vi "TryUpdateDigitalOutputSample.vi"   [LabVIEW 2018]
uses:
  <vilib>/Platform/TimedLoop/XDataNode/timing_clust.ctl
  <vilib>/Platform/TimedLoop/XDataNode/nitl_modes.ctl
  <vilib>/Platform/TimedLoop/XDataNode/wakeup.ctl
  Telemetry/TelemetryDataTypes.ctl
  Telemetry/TelemetryUpdateModes.ctl
  Telemetry/TelemetryFields.ctl
  <vilib>/rvi/Emulation/niFpgaEmulationIsFPGAContextNoSignature.vi
  <vilib>/rvi/Emulation/niFpgaSctlEmulationGetInTimedLoop.vi
  <vilib>/rvi/errors/niFpgaSetErrorForExecOnDevCompSimple.vi
  <vilib>/rvi/eio/common/nirviEmuReportErrorAndStop.vi
  <vilib>/rvi/DataTransferAndStorage/Container/Common/niFpgaContainerGetUniqueNameForEmu.vi
  <vilib>/rvi/FIFO/Fifo_Resource/nirvififoEmulationSetSize.vi
  <vilib>/rvi/FIFO/Fifo_Resource/nirviFifoEmulationQueueMgr.vi
  <instcachedir>/0/nirviFifoEmulationQueueMgr_E5CAEC123FF24DC58D834DCA3CDAA9B5.lvgen/nirviFifoEmulationQueueMgr_E5CAEC123FF24DC58D834DCA3CDAA9B5_013.vi
  <vilib>/Utility/error.llb/Clear Errors.vi
  <vilib>/rvi/FIFO/Fifo_Resource/nirvififoEmulationCreateLock.vi
  <vilib>/rvi/Emulation/niFpgaProcessEmulError.vi
  <vilib>/rvi/FIFO/Fifo_Resource/nirvififoEmulationObtainLock.vi
  <vilib>/rvi/FIFO/Fifo_Resource/nirvififoEmulationReleaseLock.vi
  <vilib>/rvi/occurrence/nirviWaitOnOccurrenceBase.vi
  <vilib>/rvi/errors/nirviReportUnexpectedCaseInternalError.vi
  <vilib>/rvi/errors/nirviReportUnexpectedCaseInternalError (U32).vi
  <vilib>/rvi/Emulation/niFpgaEmulationReportErrorSimple.vi
  <vilib>/rvi/Emulation/niFpgaGetClockAttributes.vi
  <vilib>/rvi/Emulation/niFpgaCriticalErrorInLSC.vi
  <instcachedir>/0/nirviFifoEmulationQueueMgr_E5CAEC123FF24DC58D834DCA3CDAA9B5.lvgen/nirviFifoEmulationQueueMgr_E5CAEC123FF24DC58D834DCA3CDAA9B5_007.vi
  <vilib>/rvi/FIFO/Fifo_Resource/nirvififoEmulationDetermineInputValidOut.vi
  <vilib>/rvi/Memory/Memory_Emulation/niFpgaMemoryEmulationCacheClearOnFirstRun.vi
  <vilib>/rvi/Memory/Memory_Emulation/nirvimemoryEmulationManagerCache_MakeExclusive.vi
  <vilib>/rvi/Memory/Memory_Emulation/niFpgaMemoryEmulationValidateCache.vi
  <vilib>/rvi/Memory/Memory_Emulation/nirvimemoryEmulationManagerCache_InsertValue.vi
  <vilib>/rvi/Memory/Memory_Emulation/nirvimemoryEmulationManagerCache_ReleaseExclusive.vi
  <vilib>/rvi/Memory/Memory_Emulation/nirvimemoryEmulationManagerCache_GetValue.vi
  <vilib>/rvi/Memory/Memory_Emulation/nirvimemoryEmulationManagerCache_SetValue.vi
  <instcachedir>/0/nirviFifoEmulationQueueMgr_E5CAEC123FF24DC58D834DCA3CDAA9B5.lvgen/nirviFifoEmulationQueueMgr_E5CAEC123FF24DC58D834DCA3CDAA9B5_002.vi
  <vilib>/rvi/DataTransferAndStorage/Container/XNode/niFpgaContainer.xnode
  <vilib>/rvi/FIFO/Fifo_Resource/nirvififoEmulationRead.vi
  <vilib>/Platform/TimedLoop/XDataNode/XDataNode.xnode
  <vilib>/rvi/FIFO/Fifo_Resource/nirvififoEmulationWrite.vi
  <vilib>/rvi/DataTransferAndStorage/Register/Emulation/niFpgaRegisterEmulation.vi
  <vilib>/Platform/TimedLoop/XDataNode/XDNodeRunTimeDep.lvlib
types:
  T1 = cluster{"Sample":u64, "Timestamp":u64, "Value":u16}
  T2 = typedef "TelemetryFields.ctl" = enum16{"None", "InclinometerTxBytes", "InclinometerRxBytes", "InclinometerTxFrames", "InclinometerRxFrames", "InclinometerErrorTimestamp", "InclinometerErrorCode", "InclinometerSampleTimestamp", "InclinometerAngleRaw", "DisplacementTxBytes", "DisplacementRxBytes", "DisplacementTxFrames", "DisplacementRxFrames", "DisplacementErrorTimestamp", "DisplacementErrorCode", "DisplacementSampleTimestamp", "DisplacementRaw1", "DisplacementRaw2", "DisplacementRaw3", "DisplacementRaw4", "DisplacementRaw5", "DisplacementRaw6", "DisplacementRaw7", "DisplacementRaw8", "AccelerometerSampleCount", "AccelerometerSampleTimestamp", "AccelerometerRaw1", "AccelerometerRaw2", "AccelerometerRaw3", "AccelerometerRaw4", "AccelerometerRaw5", "AccelerometerRaw6", "AccelerometerRaw7", "AccelerometerRaw8", "GyroTxBytes", "GyroRxBytes", "GyroTxFrames", "GyroRxFrames", "GyroErrorTimestamp", "GyroErrorCode", "GyroSampleTimestamp", "GyroRawX", "GyroRawY", "GyroRawZ", "GyroStatus", "GyroSequenceNumber", "GyroTemperature", "GyroBITTimestamp", "GyroBIT0", "GyroBIT1", "GyroBIT2", "GyroBIT3", "GyroBIT4", "GyroBIT5", "GyroBIT6", "GyroBIT7", "DigitalInputSampleCount", "DigitalInputTimestamp", "DigitalInputStates", "DigitalOutputSampleCount", "DigitalOutputTimestamp", "DigitalOutputStates", "PowerSupplySampleCount", "PowerSupplyTimestamp", "PowerSupplyStates", "Modbus1ErrorFlags", "Modbus1TxByteCount", "Modbus1TxFrameCount", "Modbus1RxByteCount", "Modbus1RxFrameCount", "Modbus2ErrorFlags", "Modbus2TxByteCount", "Modbus2TxFrameCount", "Modbus2RxByteCount", "Modbus2RxFrameCount", "Modbus3ErrorFlags", "Modbus3TxByteCount", "Modbus3TxFrameCount", "Modbus3RxByteCount", "Modbus3RxFrameCount", "Modbus4ErrorFlags", "Modbus4TxByteCount", "Modbus4TxFrameCount", "Modbus4RxByteCount", "Modbus4RxFrameCount"}
  T3 = typedef "TelemetryUpdateModes.ctl" = enum8{"=", "+", "-", "|"}
  T4 = typedef "TelemetryDataTypes.ctl" = enum8{"U8", "U16", "U32", "U64", "I8", "I16", "I32", "I64", "SGL"}
  T5 = typedef "XDNodeRunTimeDep.lvlib/timing_clust.ctl" = cluster{"Expected End [f-1]":u64, "Actual End [f-1]":u64, "Finished Late? [f-1]":bool, "Expected End [i-1]":u64, "Actual End [i-1]":u64, "Finished Late? [i-1]":bool, "Expected Start [i]":u64, "Actual Start [i]":u64, "Expected Start [f]":u64, "Actual Start [f]":u64, "Source Name":string, "Structure Name":string, "Period":i64, "Deadline":i64, "Offset":i64, "Start":i64, "Priority":i32, "Timeout":i32, "Mode":T6, "Wakeup Reason":T7, "Error":errorcluster, "Source Type":string, "Secondary Source Type":string, "Global End Time":u64, "Global Start Time":u64, "Frame Duration":u64, "Iteration Duration":u64, "Assigned CPU":i32, "I/O Scan Engine Mode":u32}
  T6 = typedef "XDNodeRunTimeDep.lvlib/nitl_modes.ctl" = enum32{"No Change", "Process missed periods, maintain original phase", "Discard missed periods, maintain original phase", "Process missed periods, ignore original phase", "Discard missed periods, ignore original phase"}
  T7 = typedef "XDNodeRunTimeDep.lvlib/wakeup.ctl" = enum32{"Normal", "Aborted", "Asynchronous wakeup", "Timing source error", "Timed loop error", "Timeout"}
  T8 = typedef "TelemetryUpdateData.ctl" = cluster{"DataType":T4, "Mode":T3, "Field":T2, "Data":u64}
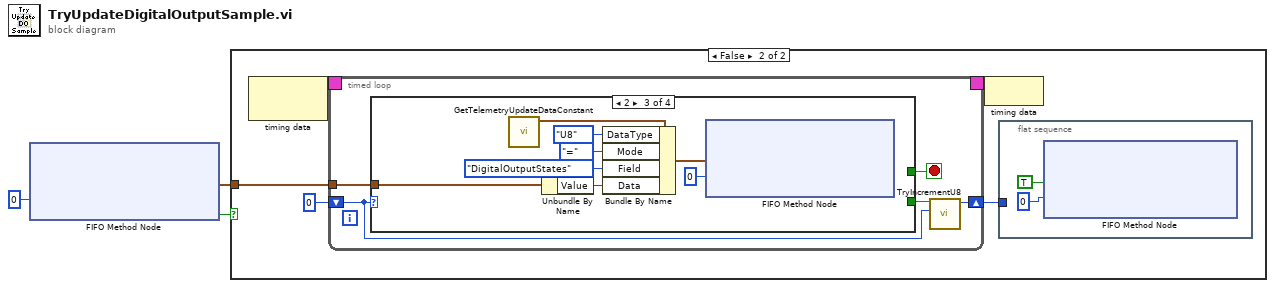
[diagram p0: block diagram]
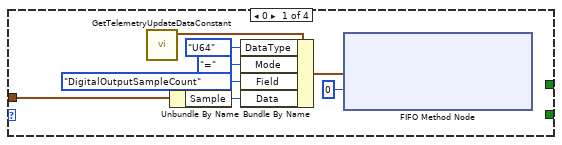
[diagram p3: hidden frame]
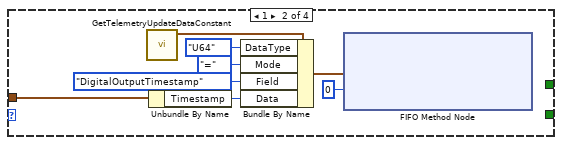
[diagram p4: hidden frame]
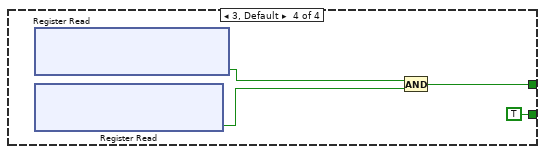
[diagram p5: hidden frame]
diagram:
  n1 = xnode ("FIFO Method Node")("Timeout"=0) -> ("Element"=w2:T1, "Timed Out?"=w3:bool)  [unwired: 1 in, 1 out]
  n2 = case shown="False" w3 {
    tunnel: w2 -> [_ w8]
    frame True {
    }
    frame False {
      n3 = node-c288() -> (w7:T5)  [unwired: 1 in]
      n4 = timed-loop {
        tunnel: w8 -> [w13]
        timing: w7 -> [_]
        timing-out: [_] -> w6
        shift-right: [w11] -> w4
        shift-left: u8 0 -> [w10]
        stop <- w12 stop-if-true
        # "Move Data to Memory"
        n5 = case shown="2" w10 {
          tunnel: w13 -> [w15 w23 w31 _]
          tunnel: [_ _ _ w41] -> w12
          tunnel: [_ _ _ TRUE] -> w9
          frame 0 {
            n6 = call "GetTelemetryUpdateDataConstant.vi"() -> ("TelemetryUpdateData"=w21:T8)  [unwired: 11 in]
            n7 = Unbundle By Name(w15) -> ("Sample"=w14:u64)
            n8 = Bundle By Name(cluster=w21, "DataType"=TelemetryDataTypes."U64" ("TelemetryDataTypes"), "Mode"=TelemetryUpdateModes."=" ("TelemetryUpdateModes"), "Field"=TelemetryFields."DigitalOutputSampleCount" ("TelemetryFields"), "Data"=w14) -> (w19:T8)
            n9 = xnode ("FIFO Method Node")("Element"=w19, "Timeout"=0) -> ()  [unwired: 1 in, 2 out]
          }
          frame 1 {
            n10 = call "GetTelemetryUpdateDataConstant.vi"() -> ("TelemetryUpdateData"=w29:T8)  [unwired: 11 in]
            n11 = Unbundle By Name(w23) -> ("Timestamp"=w22:u64)
            n12 = Bundle By Name(cluster=w29, "DataType"=TelemetryDataTypes."U64" ("TelemetryDataTypes"), "Mode"=TelemetryUpdateModes."=" ("TelemetryUpdateModes"), "Field"=TelemetryFields."DigitalOutputTimestamp" ("TelemetryFields"), "Data"=w22) -> (w27:T8)
            n13 = xnode ("FIFO Method Node")("Element"=w27, "Timeout"=0) -> ()  [unwired: 1 in, 2 out]
          }
          frame 2 {
            n14 = call "GetTelemetryUpdateDataConstant.vi"() -> ("TelemetryUpdateData"=w37:T8)  [unwired: 11 in]
            n15 = Unbundle By Name(w31) -> ("Value"=w30:u16)
            n16 = Bundle By Name(cluster=w37, "DataType"=TelemetryDataTypes."U8" ("TelemetryDataTypes"), "Mode"=TelemetryUpdateModes."=" ("TelemetryUpdateModes"), "Field"=TelemetryFields."DigitalOutputStates" ("TelemetryFields"), "Data"=w30) -> (w35:T8)
            n17 = xnode ("FIFO Method Node")("Element"=w35, "Timeout"=0) -> ()  [unwired: 1 in, 2 out]
          }
          frame 3, Default {
            n18 = xnode ("Register Read")() -> ("Data"=w39:bool)  [unwired: 1 in, 1 out]
            n19 = xnode "Register Read"() -> ("Data"=w40:bool)  [unwired: 1 in, 1 out]
            n20 = And(x=w39, y=w40) -> (x .and. y?=w41:bool)
          }
        }
        n21 = call "TryIncrementU8.vi"("In"=w10, "DontInc"=w9) -> ("Out"=w11:u8)  [unwired: 9 in]
      }
      n22 = node-c288(w6) -> ()
      n23 = flat-sequence {
        tunnel: w4 -> [_]
        frame #0 {
          n24 = xnode ("FIFO Method Node")("Element"=TRUE, "Timeout"=0) -> ()  [unwired: 1 in, 2 out]
        }
      }
    }
  }
